vi "Store Last Deployed.vi"(8 "error in (no error)":errorcluster, 9 "PicoG-Core:DeployResource":refnum<class "DeployResource.lvclass">, 10 "PicoG-Core:DeployTarget":refnum<class "DeployTarget.lvclass">, 11 "TargetPluginManager in":refnum<class "TargetPluginManager.lvclass">) -> (0 "error out":errorcluster, 3 "TargetPluginManager out":refnum<class "TargetPluginManager.lvclass">)   [LabVIEW 2020, in "PicoG-Core.lvlib" / "TargetPluginManager.lvclass"]
uses:
  TargetPluginManager.lvclass
  DeployTarget/DeployTarget.lvclass
  DeployResource/DeployResource.lvclass
  TargetPluginManager.lvclass/TargetPluginManager.ctl
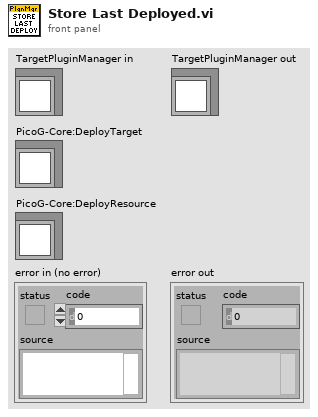
[diagram p1: front panel]
types:
  T1 = typedef "PicoG-Core.lvlib/TargetPluginManager.lvclass/Ref Data.ctl" = cluster{"Targets":refnum<class "DeployTarget.lvclass">[], "Last Target":refnum<class "DeployTarget.lvclass">, "Last Resource":refnum<class "DeployResource.lvclass">}
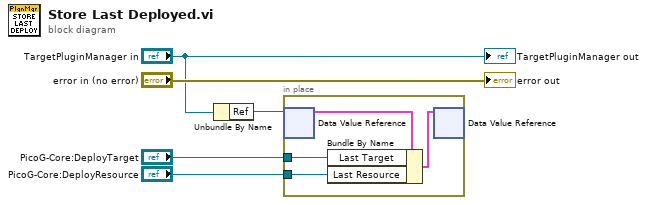
[diagram p0: block diagram]
diagram:
  n1 = Unbundle By Name("TargetPluginManager in") -> ("Ref"=w4:refnum<data-value>)
  n2 = in-place {
    in-place-border: "PicoG-Core:DeployTarget" -> [w7]
    in-place-border: "PicoG-Core:DeployResource" -> [w6]
    n3 = in-place-dvr #1(w4) -> (w9:T1)  [unwired: 1 out]
    n4 = Bundle By Name(cluster=w9, "Last Target"=w7, "Last Resource"=w6) -> (w8:T1)
    n5 = in-place-dvr #1(w8) -> ()  [unwired: 2 out]
  }
  "error out" <- "error in (no error)"
  "TargetPluginManager out" <- "TargetPluginManager in"
